vi "DI Waveform to Data UI.vi"(11 "DI Data in":digitalwaveform[](array[waveform])) -> (3 "Array":bool[](array[boolean]))   [LabVIEW 2022 SP3]
uses:
  <vilib>/Waveform/DTblOps.llb/DTbl Digital to Boolean Array.vi
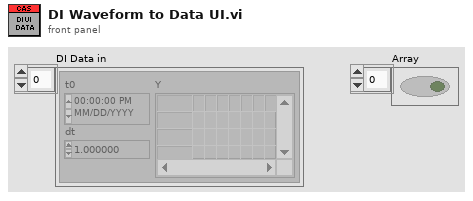
[diagram p1: front panel]
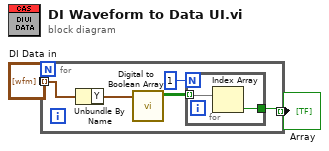
[diagram p0: block diagram]
diagram:
  n1 = for {
    tunnel: "DI Data in" -> [w7] mode=indexing
    tunnel: [w4] -> w1 mode=indexing
    n2 = Unbundle By Name(w7) -> ("Y"=w6:digitaldata)
    n3 = call-poly <vilib>:"Digital to Boolean Array.vi"("digital data"=w6) -> ("boolean array"=w5:bool[][])  [unwired: 9 in, 1 out]
    n4 = for {
      N: 1 -> [_]
      tunnel: w5 -> [w9] mode=indexing
      tunnel: [w8] -> w4
      n5 = Index Array(array=w9) -> (element=w8:bool)  [unwired: 1 in]
    }
  }
  "Array" <- w1
